vi "Update Scale.vi"(10 "Scale":dbl, 11 "References in":T1) -> (0 "error out":errorcluster)   [LabVIEW 2021, in "Multiplexer editor node.lvclass"]
uses:
  Multiplexer editor node.lvclass
  <vilib>/NI/DCAF/Tag Editor Core/Table API/Table Manager/object ref.ctl
  <vilib>/NI/DCAF/Tag Editor Core/Configuration Editor/Classes/Engine Parent/Engine Parent Editor Node.lvclass
  <vilib>/NI/DCAF/Tag Editor Core/Configuration Editor/Classes/Module editor node/module editor node.lvclass
  C:/Program Files (x86)/National Instruments/LabVIEW 2021/vi.lib/NI/Configuration Framework/serializable node/NISE_CEF_serializable node.lvclass
  configuration/Multiplexer configuration.lvclass
  C:/Program Files (x86)/National Instruments/LabVIEW 2021/vi.lib/NI/Configuration Framework/serializable configuration/NISE_CEF_serializable configuration.lvclass
  configuration/Multiplexer configuration.lvclass/Multiplexer configuration.ctl
  configuration/Write Scale.vi
  <vilib>/NI/Configuration Framework/serializable configuration/NISE_CEF_serializable configuration.lvclass
  <vilib>/NI/DCAF/Tag Editor Core/Table API/Table Manager/Table Manager.lvclass
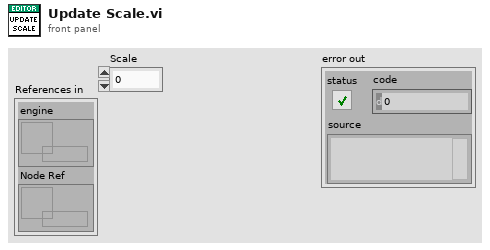
[diagram p1: front panel]
types:
  T1 = typedef "Table Manager.lvlib/Table Manager.lvclass/object ref.ctl" = cluster{"engine":refnum<data-value>, "Node Ref":refnum<data-value>}
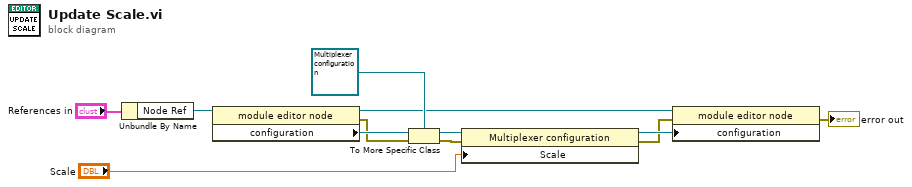
[diagram p0: block diagram]
diagram:
  n1 = Unbundle By Name("References in") -> ("Node Ref"=w11:refnum<data-value>)
  n2 = property class="module editor node"(reference=w11) -> (reference out=w4:refnum<data-value>, error out=w6:errorcluster, "configuration"=w10:refnum<class "NISE_CEF_serializable configuration.lvclass">)  [unwired: 1 in]
  n3 = To More Specific Class(target class=refnum<class "Multiplexer configuration.lvclass"> refnum ("Multiplexer configuration"), reference=w10, error in=w6) -> (specific class reference=w8:refnum<class "Multiplexer configuration.lvclass">, error out=w7:errorcluster)
  n4 = property class="Multiplexer configuration"(reference=w8, error in=w7, "Scale"="Scale") -> (reference out=w3:refnum<class "Multiplexer configuration.lvclass">, error out=w2:errorcluster)
  n5 = property class="module editor node"(reference=w4, error in=w2, "configuration"=w3) -> (error out=→"error out":errorcluster)  [unwired: 1 out]
